vi "HEUI_LEDs to HEUI_Display.vi"(7 "HEUI_LEDs":T8) -> (8 "HEUI_Display":T1)   [LabVIEW 2016, in "TL27.lvlib"]
uses:
  Projects/TL27.lvlib
  controls/HEUI_LEDs.ctl
  controls/HEUI_Display.ctl
  controls/Cycle Selection Enum.ctl
  controls/Stain Enum.ctl
  controls/Temp Enum.ctl
  controls/Soil Enum.ctl
  controls/Spin Enum.ctl
  controls/750 Status Enum.ctl
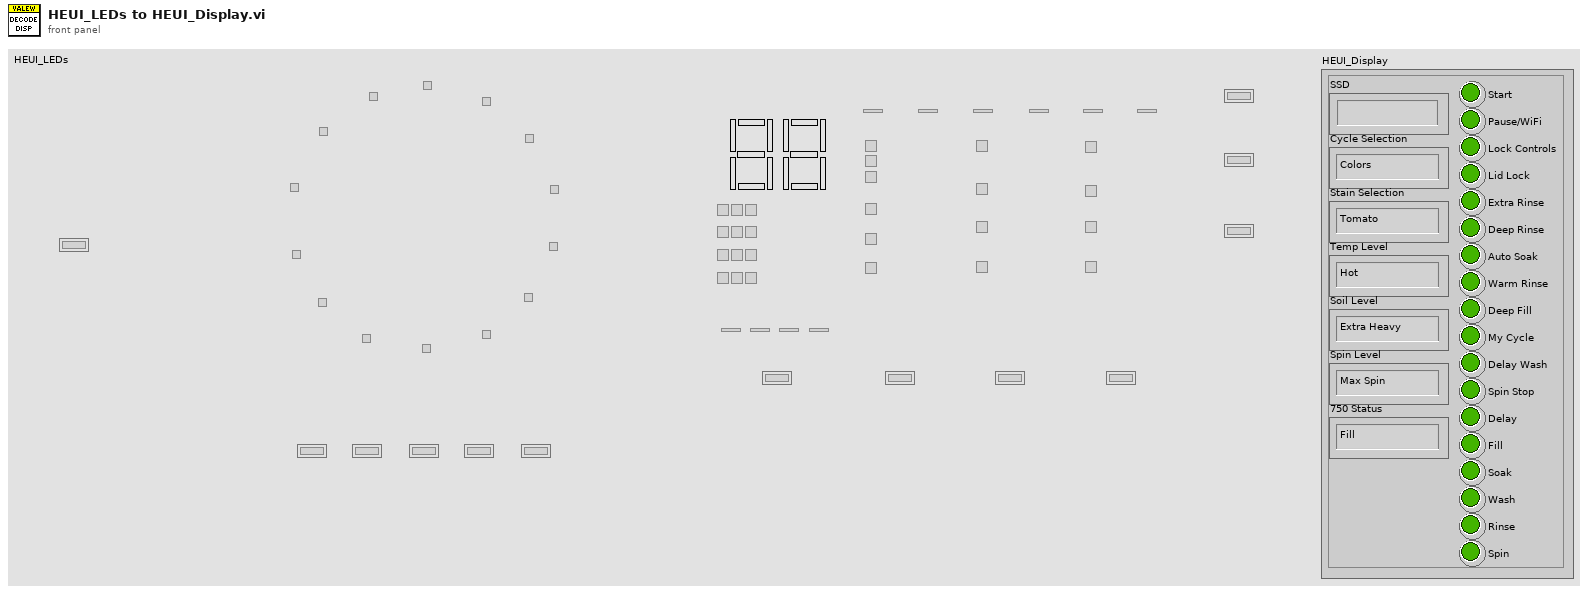
[diagram p1: front panel]
types:
  T1 = typedef "TL27.lvlib/HEUI_Display.ctl" = cluster{"SSD":string, "Cycle Selection":T2, "Stain Selection":T3, "Temp Level":T4, "Soil Level":T5, "Spin Level":T6, "750 Status":T7, "Start":bool, "Pause/WiFi":bool, "Lock Controls":bool, "Lid Lock":bool, "Extra Rinse":bool, "Deep Rinse":bool, "Auto Soak":bool, "Warm Rinse":bool, "Deep Fill":bool, "My Cycle":bool, "Delay Wash":bool, "Spin Stop":bool, "Delay":bool, "Fill":bool, "Soak":bool, "Wash":bool, "Rinse":bool, "Spin":bool}
  T2 = typedef "TL27.lvlib/Cycle Selection Enum.ctl" = enum16{"Colors", "Easy Care", "Delicates", "Hand Wash", "Active Wear", "Speed Wash", "Rinse and Spin", "Drain and Spin", "Basket Clean", "Jeans", "Heavy Duty", "Bulky Items", "Towels", "Whites", "Off", "*Incorrect*"}
  T3 = typedef "TL27.lvlib/Stain Enum.ctl" = enum16{"Tomato", "Wine", "Blood", "Grass", "Dirt", "Off", "*Incorrect*"}
  T4 = typedef "TL27.lvlib/Temp Enum.ctl" = enum16{"Hot", "Warm", "Colors", "Cool", "Cold", "Tap Cold", "Off", "*Incorrect*"}
  T5 = typedef "TL27.lvlib/Soil Enum.ctl" = enum16{"Extra Heavy", "Heavy", "Normal", "Light", "Off", "*Incorrect*"}
  T6 = typedef "TL27.lvlib/Spin Enum.ctl" = enum16{"Max Spin", "More Spin", "Normal Spin", "No Spin", "Off", "*Incorrect*"}
  T7 = typedef "TL27.lvlib/750 Status Enum.ctl" = enum16{"Fill", "Wash", "Rinse", "Spin", "Off", "*Incorrect*"}
  T8 = typedef "TL27.lvlib/HEUI_LEDs.ctl" = cluster{"Z101 - Start":bool, "Z103 - Colors":bool, "Z104 - Whites":bool, "Z105 - Towels":bool, "Z106 - Bulky Items":bool, "Z107 - Heavy Duty":bool, "Z108 - Jeans":bool, "Z109 - Basket Clean":bool, "Z110 - Drain and Spin":bool, "Z111 - Rinse and Spin":bool, "Z112 - Speed Wash":bool, "Z113 - Active Wear":bool, "Z114 - Hand Wash":bool, "Z115 - Delicates":bool, "Z116 - Easy Care":bool, "Z117 - Tomato":bool, "Z118 - Wine":bool, "Z119 - Blood":bool, "Z120 - Grass":bool, "Z121 - Dirt":bool, "Z122_MSB_A":bool, "Z123_MSB_B":bool, "Z124_MSB_G":bool, "Z125_MSB_C":bool, "Z126_MSB_D":bool, "Z127_MSB_E":bool, "Z128_MSB_F":bool, "Z129_LSB_A":bool, "Z130_LSB_B":bool, "Z131_LSB_G":bool, "Z132_LSB_C":bool, "Z133_LSB_D":bool, "Z134_LSB_E":bool, "Z135_LSB_F":bool, "Z136 - Pause":bool, "Z137 - Pause":bool, "Z138 - Lock Controls":bool, "Z139 - Lock Controls":bool, "Z140 - Lock Controls":bool, "Z141 - Lid Lock":bool, "Z142 - Lid Lock":bool, "Z143 - Lid Lock":bool, "Z144 - Good":bool, "Z145":bool, "Z146":bool, "Z147 - Better":bool, "Z148 - Delay":bool, "Z149 - Fill":bool, "Z150 - Soak":bool, "Z151 - Wash":bool, "Z152 - Rinse":bool, "Z153 - Spin":bool, "Z154 - Hot":bool, "Z155 - Warm":bool, "Z156 - Colors":bool, "Z157 - Cool":bool, "Z158 - Cold":bool, "Z159 - Tap Cold":bool, "Z160 - Extra Heavy":bool, "Z161 - Heavy":bool, "Z162 - Normal":bool, "Z163 - Light":bool, "Z164 - Max Spin":bool, "Z165 - More Spin":bool, "Z166 - Normal Spin":bool, "Z167 - No Spin":bool, "Z168 - Extra Rinse":bool, "Z170 - Deep Rinse":bool, "Z171 - Auto Soak":bool, "Z172 - Warm Rinse":bool, "Z173 - Deep Fill":bool, "Z174 - My Cycles":bool, "Z175 - Delay Wash":bool, "Z176 - Spin Stop":bool, "Z177 - Spin Stop":bool, "Z178 - Spin Stop":bool, "Z179 - Pause":bool, "Z109":bool, "Z110":bool, "Z123":bool, "Z124":bool, "Z140":bool, "Unused0":bool, "Unused1":bool, "Unused2":bool, "Unused3":bool, "Channel_Off":bool, "Channel_Cycle_Unmapped":bool}
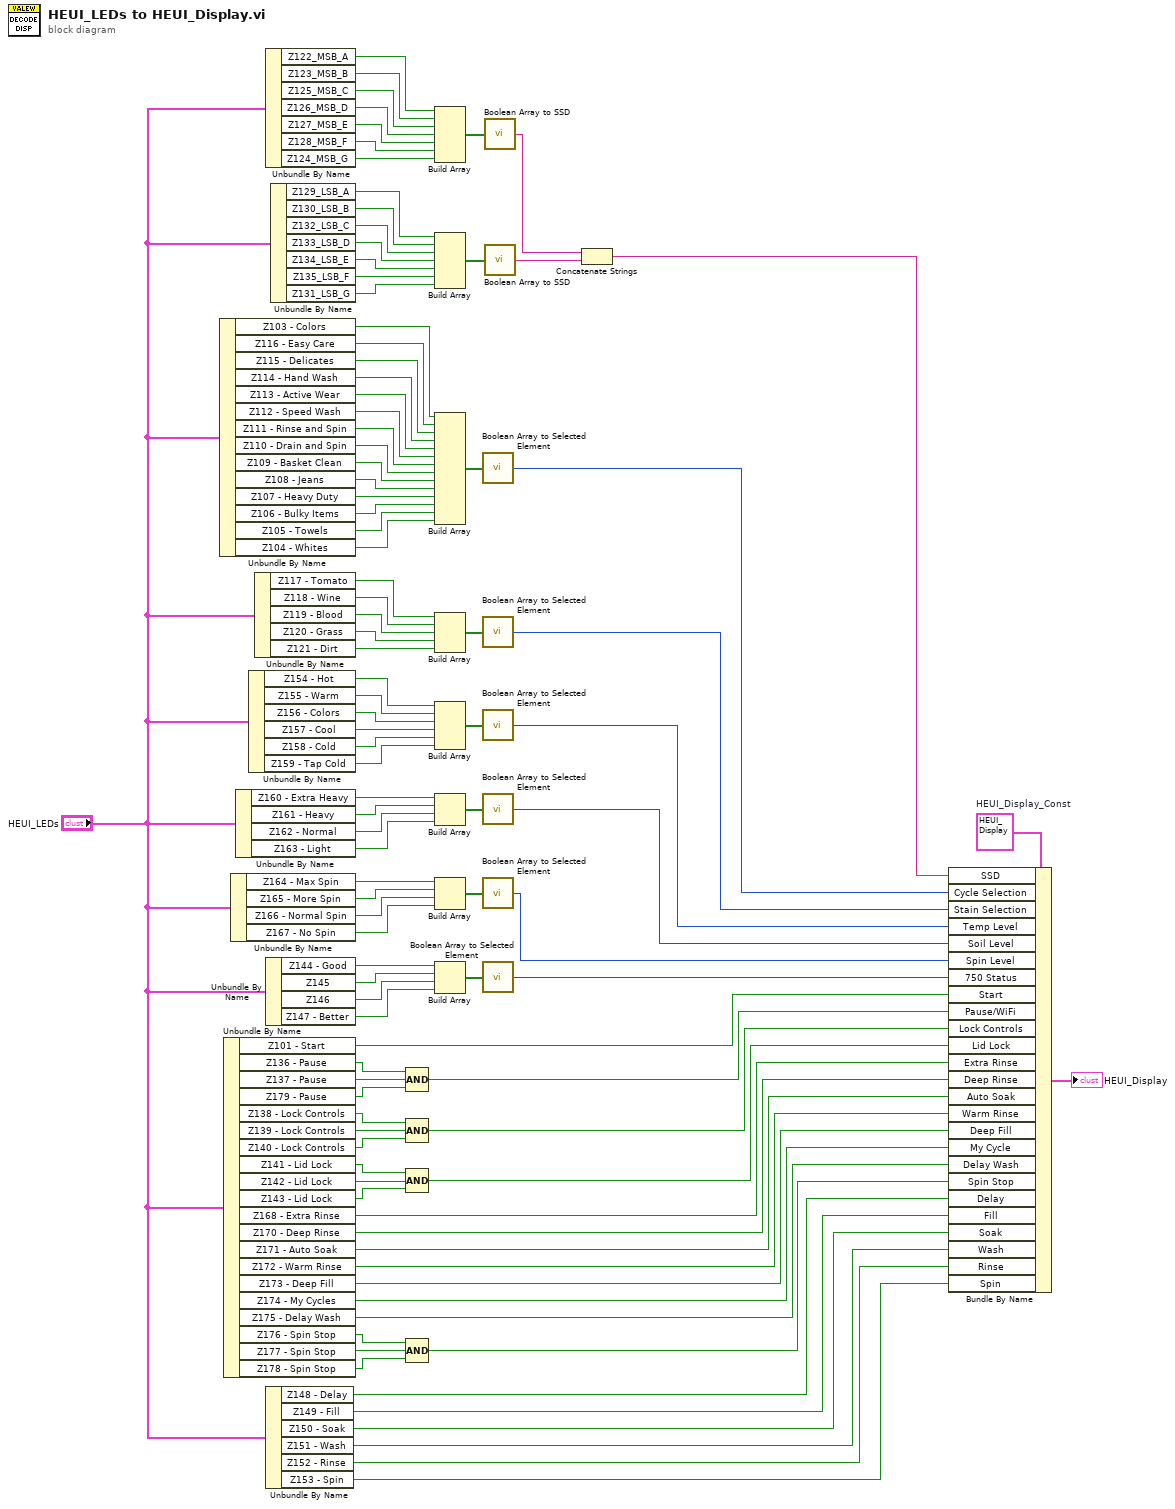
[diagram p0: block diagram]
diagram:
  w28 = T1 {"SSD"="", "Cycle Selection"=enum."Colors", "Stain Selection"=enum."Tomato", "Temp Level"=enum."Hot", "Soil Level"=enum."Extra Heavy", "Spin Level"=enum."Max Spin", "750 Status"=enum."Fill", "Start"=FALSE, "Pause/WiFi"=FALSE, "Lock Controls"=FALSE, "Lid Lock"=FALSE, "Extra Rinse"=FALSE, "Deep Rinse"=FALSE, "Auto Soak"=FALSE, "Warm Rinse"=FALSE, "Deep Fill"=FALSE, "My Cycle"=FALSE, "Delay Wash"=FALSE, "Spin Stop"=FALSE, "Delay"=FALSE, "Fill"=FALSE, "Soak"=FALSE, "Wash"=FALSE, "Rinse"=FALSE, "Spin"=FALSE}  # HEUI_Display_Const
  n1 = Unbundle By Name("HEUI_LEDs") -> ("Z103 - Colors"=w83:bool, "Z116 - Easy Care"=w82:bool, "Z115 - Delicates"=w81:bool, "Z114 - Hand Wash"=w80:bool, "Z113 - Active Wear"=w79:bool, "Z112 - Speed Wash"=w78:bool, "Z111 - Rinse and Spin"=w77:bool, "Z110 - Drain and Spin"=w76:bool, "Z109 - Basket Clean"=w75:bool, "Z108 - Jeans"=w74:bool, "Z107 - Heavy Duty"=w73:bool, "Z106 - Bulky Items"=w72:bool, "Z105 - Towels"=w71:bool, "Z104 - Whites"=w70:bool)
  n2 = Unbundle By Name("HEUI_LEDs") -> ("Z101 - Start"=w26:bool, "Z136 - Pause"=w40:bool, "Z137 - Pause"=w39:bool, "Z179 - Pause"=w38:bool, "Z138 - Lock Controls"=w37:bool, "Z139 - Lock Controls"=w36:bool, "Z140 - Lock Controls"=w35:bool, "Z141 - Lid Lock"=w34:bool, "Z142 - Lid Lock"=w33:bool, "Z143 - Lid Lock"=w32:bool, "Z168 - Extra Rinse"=w22:bool, "Z170 - Deep Rinse"=w21:bool, "Z171 - Auto Soak"=w20:bool, "Z172 - Warm Rinse"=w19:bool, "Z173 - Deep Fill"=w18:bool, "Z174 - My Cycles"=w17:bool, "Z175 - Delay Wash"=w16:bool, "Z176 - Spin Stop"=w31:bool, "Z177 - Spin Stop"=w30:bool, "Z178 - Spin Stop"=w29:bool)
  n3 = Unbundle By Name("HEUI_LEDs") -> ("Z164 - Max Spin"=w49:bool, "Z165 - More Spin"=w48:bool, "Z166 - Normal Spin"=w47:bool, "Z167 - No Spin"=w46:bool)
  n4 = Unbundle By Name("HEUI_LEDs") -> ("Z160 - Extra Heavy"=w55:bool, "Z161 - Heavy"=w54:bool, "Z162 - Normal"=w53:bool, "Z163 - Light"=w52:bool)
  n5 = Unbundle By Name("HEUI_LEDs") -> ("Z154 - Hot"=w62:bool, "Z155 - Warm"=w61:bool, "Z156 - Colors"=w60:bool, "Z157 - Cool"=w59:bool, "Z158 - Cold"=w58:bool, "Z159 - Tap Cold"=w57:bool)
  n6 = Unbundle By Name("HEUI_LEDs") -> ("Z117 - Tomato"=w69:bool, "Z118 - Wine"=w68:bool, "Z119 - Blood"=w67:bool, "Z120 - Grass"=w66:bool, "Z121 - Dirt"=w65:bool)
  n7 = Unbundle By Name("HEUI_LEDs") -> ("Z122_MSB_A"=w101:bool, "Z123_MSB_B"=w100:bool, "Z125_MSB_C"=w99:bool, "Z126_MSB_D"=w98:bool, "Z127_MSB_E"=w97:bool, "Z128_MSB_F"=w96:bool, "Z124_MSB_G"=w95:bool)
  n8 = Unbundle By Name("HEUI_LEDs") -> ("Z144 - Good"=w44:bool, "Z145"=w43:bool, "Z146"=w42:bool, "Z147 - Better"=w41:bool)
  n9 = Unbundle By Name("HEUI_LEDs") -> ("Z148 - Delay"=w6:bool, "Z149 - Fill"=w5:bool, "Z150 - Soak"=w4:bool, "Z151 - Wash"=w3:bool, "Z152 - Rinse"=w2:bool, "Z153 - Spin"=w1:bool)
  n10 = Unbundle By Name("HEUI_LEDs") -> ("Z129_LSB_A"=w94:bool, "Z130_LSB_B"=w93:bool, "Z132_LSB_C"=w92:bool, "Z133_LSB_D"=w91:bool, "Z134_LSB_E"=w90:bool, "Z135_LSB_F"=w89:bool, "Z131_LSB_G"=w88:bool)
  n11 = Compound Arithmetic op=AND(w40, w39, w38) -> (w25:bool)
  n12 = Compound Arithmetic op=AND(w37, w36, w35) -> (w24:bool)
  n13 = Compound Arithmetic op=AND(w34, w33, w32) -> (w23:bool)
  n14 = Compound Arithmetic op=AND(w31, w30, w29) -> (w15:bool)
  n15 = Build Array(w101, w100, w99, w98, w97, w96, w95) -> (w87:bool[])
  n16 = Build Array(w94, w93, w92, w91, w90, w89, w88) -> (w86:bool[])
  n17 = Build Array(w83, w82, w81, w80, w79, w78, w77, w76, w75, w74, w73, w72, w71, w70) -> (w63:bool[])
  n18 = Build Array(w69, w68, w67, w66, w65) -> (w64:bool[])
  n19 = Build Array(w62, w61, w60, w59, w58, w57) -> (w56:bool[])
  n20 = Build Array(w55, w54, w53, w52) -> (w51:bool[])
  n21 = Build Array(w49, w48, w47, w46) -> (w50:bool[])
  n22 = Build Array(w44, w43, w42, w41) -> (w45:bool[])
  n23 = call "Boolean Array to Selected Element.vi"("Bool Array In"=w63) -> ("Selected Element Out"=w9:i32)  [unwired: 14 in]
  n24 = call "Boolean Array to Selected Element.vi"("Bool Array In"=w64) -> ("Selected Element Out"=w10:i32)  [unwired: 14 in]
  n25 = call "Boolean Array to Selected Element.vi"("Bool Array In"=w56) -> ("Selected Element Out"=w14:i32)  [unwired: 14 in]
  n26 = call "Boolean Array to Selected Element.vi"("Bool Array In"=w51) -> ("Selected Element Out"=w11:i32)  [unwired: 14 in]
  n27 = call "Boolean Array to Selected Element.vi"("Bool Array In"=w50) -> ("Selected Element Out"=w12:i32)  [unwired: 14 in]
  n28 = call "Boolean Array to Selected Element.vi"("Bool Array In"=w45) -> ("Selected Element Out"=w13:i32)  [unwired: 14 in]
  n29 = call "Boolean Array to SSD.vi"("7 Segment Bool Array In"=w87) -> ("7 Segment Out"=w85:string)  [unwired: 14 in]
  n30 = call "Boolean Array to SSD.vi"("7 Segment Bool Array In"=w86) -> ("7 Segment Out"=w84:string)  [unwired: 14 in]
  n31 = Concatenate Strings(w85, w84) -> (w8:string)
  n32 = Bundle By Name(cluster=w28, "SSD"=w8, "Cycle Selection"=w9, "Stain Selection"=w10, "Temp Level"=w14, "Soil Level"=w11, "Spin Level"=w12, "750 Status"=w13, "Start"=w26, "Pause/WiFi"=w25, "Lock Controls"=w24, "Lid Lock"=w23, "Extra Rinse"=w22, "Deep Rinse"=w21, "Auto Soak"=w20, "Warm Rinse"=w19, "Deep Fill"=w18, "My Cycle"=w17, "Delay Wash"=w16, "Spin Stop"=w15, "Delay"=w6, "Fill"=w5, "Soak"=w4, "Wash"=w3, "Rinse"=w2, "Spin"=w1) -> (→"HEUI_Display":T1)
